vi "Audio.Ckeck for presense of Multi Tones.vi"(8 "Require All":bool, 9 "Tolerance(+/-%)":dbl=3.0, 10 "Stimulus Tones":T1(array[cluster])=[{"frequency"=1000.0, "amplitude"=1.0, "phase"=0.0}], 11 "Detected Tones":T2(array[cluster]) {"detected phase (deg)" format="%_6g"; "detected amplitude" format="%_6p"; "detected frequency" format="%_6p"}) -> (3 "Pass":bool)   [LabVIEW 2018]
panel:
  out "Detected":bool[](array[boolean])
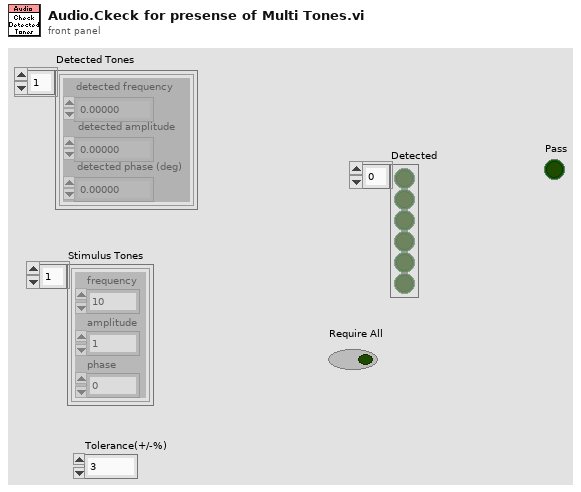
[diagram p1: front panel]
types:
  T1 = cluster{"frequency":dbl, "amplitude":dbl, "phase":dbl}[]
  T2 = cluster{"detected frequency":dbl, "detected amplitude":dbl, "detected phase (deg)":dbl}[]
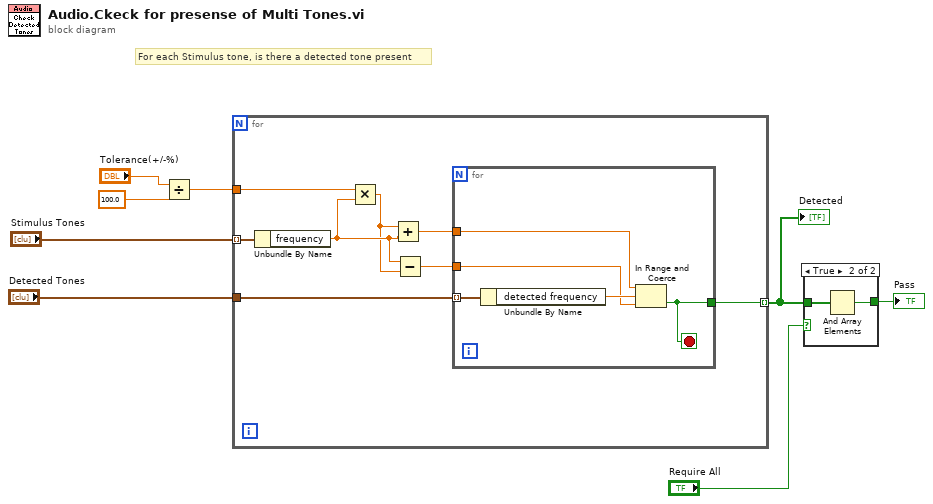
[diagram p0: block diagram]
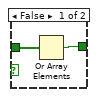
[diagram p2: hidden frame]
diagram:
  # "For each Stimulus tone, is there a detected tone present"
  n1 = Divide(x="Tolerance(+/-%)", y=100.0) -> (x/y=w4:dbl)
  n2 = for {
    tunnel: "Detected Tones" -> [w16]
    tunnel: "Stimulus Tones" -> [w15] mode=indexing
    tunnel: w4 -> [w14]
    tunnel: [w9] -> w3 mode=indexing
    n3 = Unbundle By Name(w15) -> ("frequency"=w13:dbl)
    n4 = Multiply(x=w14, y=w13) -> (x*y=w12:dbl)
    n5 = Add(x=w12, y=w13) -> (x+y=w11:dbl)
    n6 = Subtract(x=w13, y=w12) -> (x-y=w10:dbl)
    n7 = for {
      tunnel: w16 -> [w21] mode=indexing
      tunnel: w11 -> [w19]
      tunnel: w10 -> [w18]
      tunnel: [w17] -> w9
      stop <- w17 stop-if-true
      n8 = Unbundle By Name(w21) -> ("detected frequency"=w20:dbl)
      n9 = In Range and Coerce(upper limit=w19, x=w20, lower limit=w18) -> (In Range?=w17:bool)  [unwired: 1 out]
    }
  }
  "Detected" <- w3
  n10 = case shown="True" "Require All" {
    tunnel: w3 -> [w23 w24]
    tunnel: [w22 w25] -> w2
    frame False {
      n11 = Or Array Elements(Boolean array=w23) -> (logical OR=w22:bool)
    }
    frame True {
      n12 = And Array Elements(Boolean array=w24) -> (logical AND=w25:bool)
    }
  }
  "Pass" <- w2
